vi "获取奶茶规格.vi"(10 "Folder Path":path=path "C:/Users/lenovo/Desktop/奶茶店/规格") -> (1 "清单名称":string[](array[string]), 2 "规格":refnum<class>[](array[class]))   [LabVIEW 2016, in "点单.lvclass"]
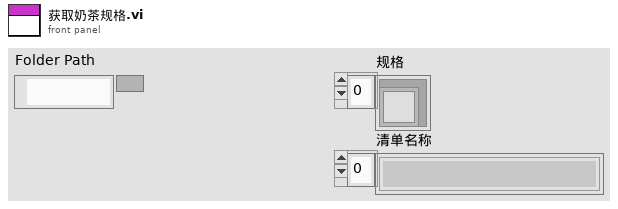
[diagram p1: front panel]
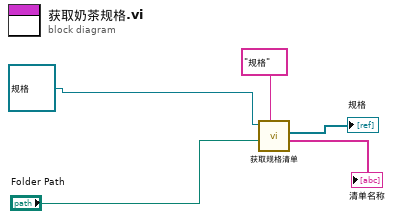
[diagram p0: block diagram]
diagram:
  n1 = call "获取规格清单.vi"("父类"="规格", "Folder Path"="Folder Path", "规格 输入"=refnum<class "规格.lvclass"> refnum ("规格.lvclass")) -> ("清单名称"=→"清单名称":string[], "规格"=→"规格":refnum<class>[])  [unwired: 5 in, 2 out]
